vi "Save Data v1.00.vi"(4 "Parameters":T1={"Magnetic Field"=0.0, "Temperature"=0.0, "Exposure Time"=0.0, "Mag ID string"="", "User Name"="", "Comments"="", "SaveComments?"=1, "X-Axis Unit"=1, "Delimitor"=0, "File Format"=0, "Sample Name"="Sample1"} {"File Format" items=["Macintosh (EOL: CR)", "Unix (EOL: LF)", "DOS/Windows (EOL: CR+LF)"]; "Delimitor" items=["TAB", "COMMA", "SPACE"]; "X-Axis Unit" items=["Point #", "nm", "eV", "meV", "cm-1"]; "SaveComments?" items=["Bare data only", "Saved in the Header Area", "Saved as a Parameter File"]; "Exposure Time" format="%.2f"; "Temperature" format="%.2f"; "Magnetic Field" format="%.2f"}, 5 "Data":dbl[][](array[numeric]) format="%.2f", 7 "File Name":string, 8 "Directory Path":path=path "/DATA") -> (0 "Final File path":path, 1 "Output File Name":string, 2 "Temperature output":dbl format="%.2f", 3 "Field output":dbl format="%.2f")   [LabVIEW 2020]
uses:
  Globals and TypeDefs/Global Varibal Control.vi
panel:
  out "Stop":bool=TRUE
  out "Contents Written":string
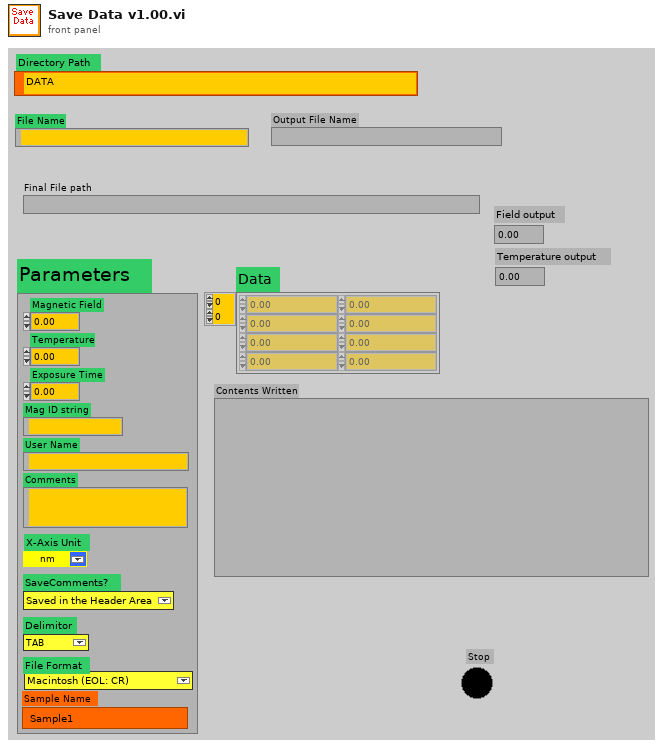
[diagram p1: front panel]
types:
  T1 = cluster{"Magnetic Field":dbl, "Temperature":dbl, "Exposure Time":dbl, "Mag ID string":string, "User Name":string, "Comments":string, "SaveComments?":u16, "X-Axis Unit":u16, "Delimitor":u16, "File Format":u16, "Sample Name":string}
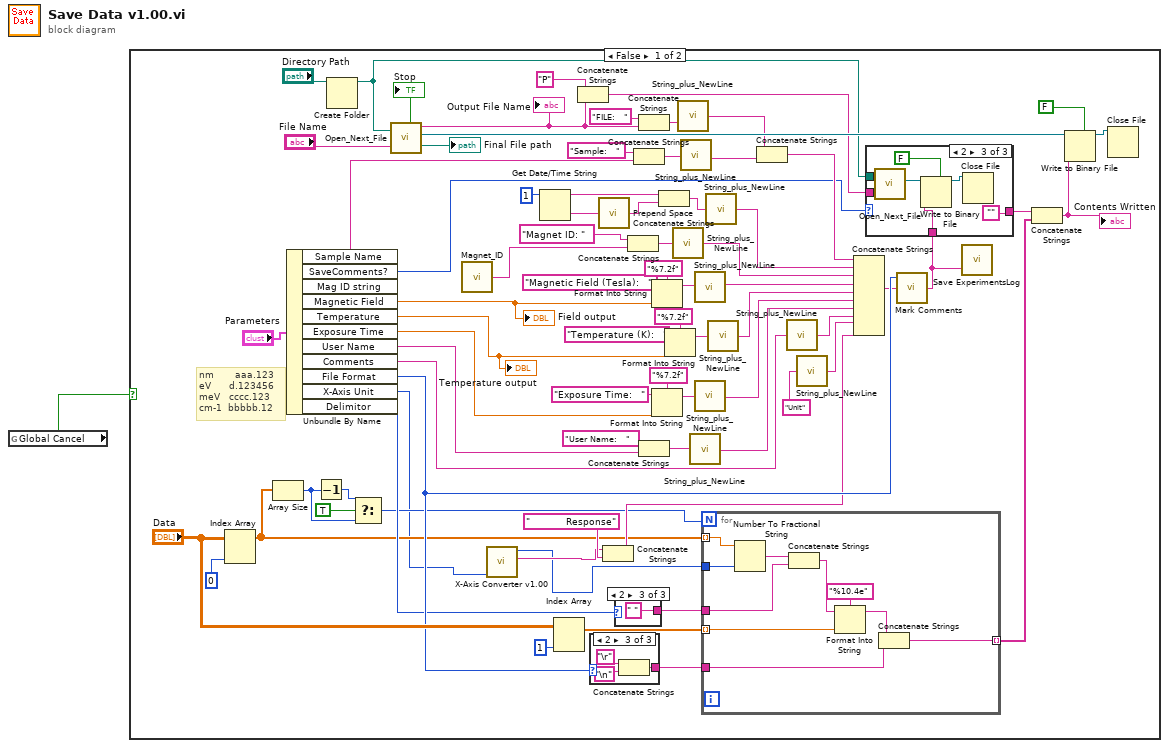
[diagram p0: block diagram]
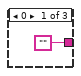
[diagram p2: hidden frame]
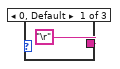
[diagram p4: hidden frame]
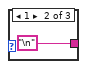
[diagram p5: hidden frame]
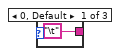
[diagram p6: hidden frame]
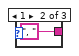
[diagram p7: hidden frame]
diagram:
  n1 = global read "Global Varibal Control.vi" "Global Cancel"() -> (w1:bool)
  n2 = case shown="False" w1 {
    frame False {
      # "nm       aaa.123\neV      d.123456\nmeV   cccc.123\ncm-1  bbbbb.12"
      n3 = Index Array(array="Data", index (col)=0) -> (element=w11:dbl[])  [unwired: 1 in]
      n4 = Array Size(array=w11) -> (size(s)=w8:i32)
      n5 = Unbundle By Name("Parameters") -> ("Sample Name"=w48:string, "SaveComments?"=w16:u16, "Magnetic Field"=w13:dbl, "Temperature"=w12:dbl, "Exposure Time"=w58:dbl, "User Name"=w57:string, "Comments"=w56:string, "File Format"=w55:u16, "X-Axis Unit"=w6:u16, "Delimitor"=w54:u16)  [unwired: 1 out]
      "Field output" <- w13
      "Temperature output" <- w12
      n6 = Decrement(x=w8) -> (x-1=w9:i32)
      n7 = Create Folder(path (use dialog)="Directory Path") -> (created path=w63:path)  [unwired: 2 in, 2 out]
      n8 = Select(t=w9, s=TRUE, f=w8) -> (s? t:f=w7:i32)
      n9 = call "Open_Next_File.vi"("Input File Pattern"="File Name", "Dir Path"=w63) -> ("Final File path"=→"Final File path":path, "File Ref Num"=w76:refnum<file>, "Output File Name"=w60:string, "Stop"=→"Stop":bool)  [unwired: 1 out]
      "Output File Name" <- w60
      n10 = call "Magnet_ID.vi"() -> ("Cell"=w3:string)
      n11 = call "X-Axis Converter v1.00.vi"("X-Axis Unit"=w6) -> ("X-Axis Unit String"=w5:string, "Precision"=w4:i32)  [unwired: 4 in, 2 out]
      n12 = Get Date/Time String(date format (0)=1) -> (date string=w41:string, time string=w43:string)  [unwired: 2 in]
      n13 = Index Array(array="Data", index (col)=1) -> (element=w69:dbl[])  [unwired: 1 in]
      n14 = Concatenate Strings("P", w60) -> (w64:string)
      n15 = case shown="2" w55 {
        tunnel: ["\r" "\n" w90] -> w67
        frame 0, Default {
        }
        frame 1 {
        }
        frame 2 {
          n16 = Concatenate Strings("\r", "\n") -> (w90:string)
        }
      }
      n17 = call "Prepend Space.vi"("Input String"=w43) -> ("Space + Input String"=w42:string)
      n18 = Concatenate Strings(w5, "            Response") -> (w52:string)
      n19 = case shown="2" w54 {
        tunnel: ["\t" ", " " "] -> w68
        frame 0, Default {
        }
        frame 1 {
        }
        frame 2 {
        }
      }
      n20 = Concatenate Strings("Magnet ID: ", w3) -> (w37:string)
      n21 = Concatenate Strings("Sample:   ", w48) -> (w49:string)
      n22 = Concatenate Strings("FILE:   ", w60) -> (w51:string)
      n23 = Concatenate Strings("User Name:   ", w57) -> (w22:string)
      n24 = Format Into String(format string="%7.2f", initial string="Magnetic Field (Tesla):   ", w13) -> (resulting string=w34:string)  [unwired: 1 in, 1 out]
      n25 = Format Into String(format string="%7.2f", initial string="Exposure Time:   ", w58) -> (resulting string=w25:string)  [unwired: 1 in, 1 out]
      n26 = Concatenate Strings(w41, w42) -> (w40:string)
      n27 = Format Into String(format string="%7.2f", initial string="Temperature (K):   ", w12) -> (resulting string=w30:string)  [unwired: 1 in, 1 out]
      n28 = call "String_plus_NewLine.vi"("Input String"=w37) -> ("Input String +[\\n]"=w36:string)
      n29 = call "String_plus_NewLine.vi"("Input String"=w51) -> ("Input String +[\\n]"=w47:string)
      n30 = call "String_plus_NewLine.vi"("Input String"=w49) -> ("Input String +[\\n]"=w46:string)
      n31 = call "String_plus_NewLine.vi"("Input String"=w22) -> ("Input String +[\\n]"=w21:string)
      n32 = call "String_plus_NewLine.vi"("Input String"=w34) -> ("Input String +[\\n]"=w29:string)
      n33 = call "String_plus_NewLine.vi"("Input String"=w25) -> ("Input String +[\\n]"=w24:string)
      n34 = for {
        N: w7 -> [_]
        tunnel: w69 -> [w100] mode=indexing
        tunnel: w11 -> [w103] mode=indexing
        tunnel: w4 -> [w104]
        tunnel: w68 -> [w102]
        tunnel: w67 -> [w97]
        tunnel: [w96] -> w53 mode=indexing
        n35 = Number To Fractional String(number=w103, precision (6)=w104) -> (F-format string=w105:string)  [unwired: 2 in]
        n36 = Concatenate Strings(w105, w102) -> (w101:string)
        n37 = Format Into String(format string="%10.4e", initial string=w101, w100) -> (resulting string=w98:string)  [unwired: 1 in, 1 out]
        n38 = Concatenate Strings(w98, w97) -> (w96:string)
      }
      n39 = call "String_plus_NewLine.vi"("Input String"=w40) -> ("Input String +[\\n]"=w39:string)
      n40 = call "String_plus_NewLine.vi"("Input String"=w30) -> ("Input String +[\\n]"=w28:string)
      n41 = Concatenate Strings(w47, w46) -> (w45:string)
      n42 = call "String_plus_NewLine.vi"("Input String"=w56) -> ("Input String +[\\n]"=w20:string)
      n43 = call "String_plus_NewLine.vi"("Input String"="Unit") -> ("Input String +[\\n]"=w19:string)
      n44 = Concatenate Strings(w45, w39, w36, w29, w28, w24, w21, w20, w19, w52) -> (w18:string)
      n45 = call "Mark Comments.vi"("Input String"=w18, "File Format"=w55) -> ("Output String"=w14:string)  [unwired: 1 in]
      n46 = case shown="2" w16 {
        tunnel: w64 -> [_ _ w87]
        tunnel: w63 -> [_ _ w86]
        tunnel: w14 -> [_ w80 w83]
        tunnel: ["" w80 ""] -> w15
        frame 0 {
        }
        frame 1, Default {
        }
        frame 2 {
          n47 = call "Open_Next_File.vi"("Input File Pattern"=w87, "Dir Path"=w86) -> ("File Ref Num"=w85:refnum<file>)  [unwired: 4 out]
          n48 = Write to Binary File(file (use dialog)=w85, data=w83, 5:FALSE ("prepend array or string size? (T)")) -> (refnum out=w84:refnum<file>)  [unwired: 3 in, 2 out]
          n49 = Close File(refnum=w84) -> ()  [unwired: 1 in, 2 out]
        }
      }
      n50 = call "Save ExperimentsLog.vi"("Contents Written"=w14) -> ()  [unwired: 2 in]
      n51 = Concatenate Strings(w15, w53) -> (w62:string)
      "Contents Written" <- w62
      n52 = Write to Binary File(file (use dialog)=w76, data=w62, 5:FALSE ("prepend array or string size? (T)")) -> (refnum out=w75:refnum<file>)  [unwired: 3 in, 2 out]
      n53 = Close File(refnum=w75) -> ()  [unwired: 1 in, 2 out]
    }
    frame True {
    }
  }
